vi "test_TCP_2_ convert_String_to_packet.vi"(11 "input_string":string) -> (2 "output_PrePacket":string, 3 "output_packet":string)   [LabVIEW 2014]
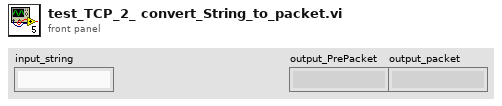
[diagram p1: front panel]
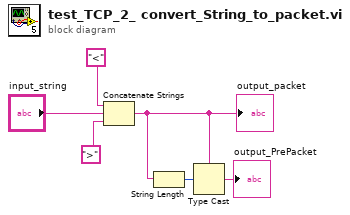
[diagram p0: block diagram]
diagram:
  n1 = Concatenate Strings("<" ("string"), "input_string", ">" ("string")) -> (w2:string)
  "output_packet" <- w2
  n2 = String Length(string=w2) -> (length=w3:i32)
  n3 = Type Cast(type=w2, x=w3) -> (*(type *) &x=→"output_PrePacket":string)
